vi "translate list to line.vi"(3 "negate y (false)":bool, 4 "distance":i32, 5 "list":cluster{"left":i32[], "right":i32[]}) -> (1 "Array":cluster{"y":i32, "x start":i32, "x end":i32}[](array[cluster]))   [LabVIEW 2009]
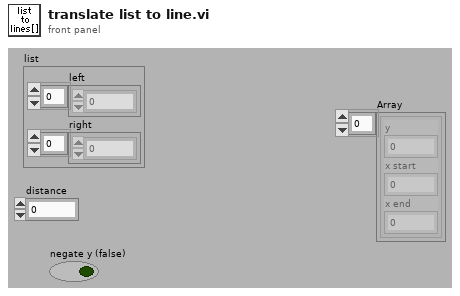
[diagram p1: front panel]
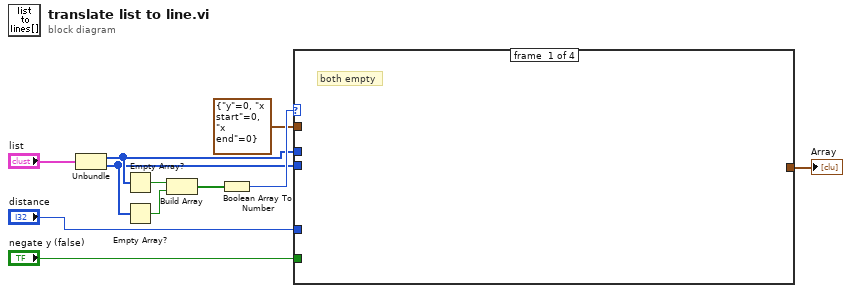
[diagram p0: block diagram]
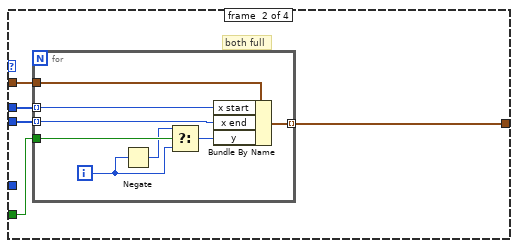
[diagram p2: hidden frame]
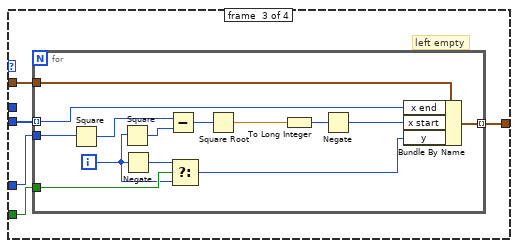
[diagram p3: hidden frame]
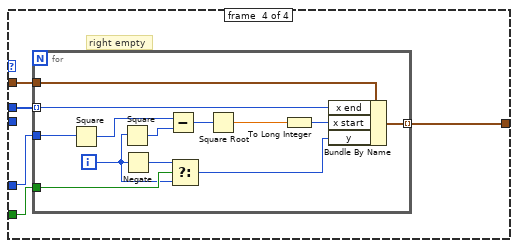
[diagram p4: hidden frame]
diagram:
  n1 = Unbundle("list") -> ("left"=w5:i32[], "right"=w4:i32[])
  n2 = Empty Array?(array=w5) -> (empty?=w9:bool)
  n3 = Empty Array?(array=w4) -> (empty?=w8:bool)
  n4 = Build Array(w9, w8) -> (w7:bool[])
  n5 = Boolean Array To Number(Boolean array=w7) -> (number=w6:u32)
  n6 = case shown="3, Default" w6 {
    tunnel: w5 -> [_ w16 _ w44]
    tunnel: w4 -> [_ w15 w28 _]
    tunnel: "negate y (false)" -> [_ w14 w26 w46]
    tunnel: cluster{"y":i32, "x start":i32, "x end":i32} {"y"=0, "x start"=0, "x end"=0} ("line") -> [_ w13 w27 w47]
    tunnel: [_ w12 w25 w45] -> w1
    tunnel: "distance" -> [_ _ w29 w48]
    frame #0 {
      # "both empty"
    }
    frame #1 {
      # "both full"
      n7 = for {
        tunnel: w16 -> [w20] mode=indexing
        tunnel: w15 -> [w21] mode=indexing
        tunnel: w14 -> [w24]
        tunnel: w13 -> [w23]
        tunnel: [w19] -> w12 mode=indexing
        i -> [w17]
        n8 = Negate(x=w17) -> (-x=w18:i32)
        n9 = Select(t=w18, s=w24, f=w17) -> (s? t:f=w22:i32)
        n10 = Bundle By Name(cluster=w23, "x start"=w20, "x end"=w21, "y"=w22) -> (w19:cluster{"y":i32, "x start":i32, "x end":i32})
      }
    }
    frame #2 {
      # "left empty"
      n11 = for {
        tunnel: w29 -> [w43]
        tunnel: w28 -> [w37] mode=indexing
        tunnel: w27 -> [w38]
        tunnel: w26 -> [w34]
        tunnel: [w30] -> w25 mode=indexing
        i -> [w32]
        n12 = Square(x=w43) -> (x^2=w41:i32)
        n13 = Square(x=w32) -> (x^2=w42:i32)
        n14 = Negate(x=w32) -> (-x=w33:i32)
        n15 = Subtract(x=w41, y=w42) -> (x-y=w40:i32)
        n16 = Select(t=w33, s=w34, f=w32) -> (s? t:f=w31:i32)
        n17 = Square Root(x=w40) -> (sqrt(x)=w39:dbl)
        n18 = To Long Integer(number=w39) -> (32bit integer=w36:i32)
        n19 = Negate(x=w36) -> (-x=w35:i32)
        n20 = Bundle By Name(cluster=w38, "x end"=w37, "x start"=w35, "y"=w31) -> (w30:cluster{"y":i32, "x start":i32, "x end":i32})
      }
    }
    frame #3 {
      # "right empty"
      n21 = for {
        tunnel: w48 -> [w61]
        tunnel: w44 -> [w55] mode=indexing
        tunnel: w47 -> [w56]
        tunnel: w46 -> [w54]
        tunnel: [w50] -> w45 mode=indexing
        i -> [w52]
        n22 = Square(x=w61) -> (x^2=w59:i32)
        n23 = Square(x=w52) -> (x^2=w60:i32)
        n24 = Negate(x=w52) -> (-x=w53:i32)
        n25 = Subtract(x=w59, y=w60) -> (x-y=w58:i32)
        n26 = Select(t=w53, s=w54, f=w52) -> (s? t:f=w51:i32)
        n27 = Square Root(x=w58) -> (sqrt(x)=w57:dbl)
        n28 = To Long Integer(number=w57) -> (32bit integer=w49:i32)
        n29 = Bundle By Name(cluster=w56, "x end"=w55, "x start"=w49, "y"=w51) -> (w50:cluster{"y":i32, "x start":i32, "x end":i32})
      }
    }
  }
  "Array" <- w1
